vi "Quick Usb Write Setting.vi"(8 "error in (no error)":errorcluster, 9 "value":u16, 10 "address":u16, 11 "hDevice":u32) -> (0 "error out":errorcluster, 2 "function return":i32, 3 "hDevice out":u32)   [LabVIEW 2011, in "QuickUSB.lvlib"]
doc: "QUSBLIB QRETURN QuickUsbWriteSetting(\n QHANDLE hDevice,\n QWORD address, \n QWORD value\n);"
uses:
  QuickUSB.lvlib
  QuickUSB.dll
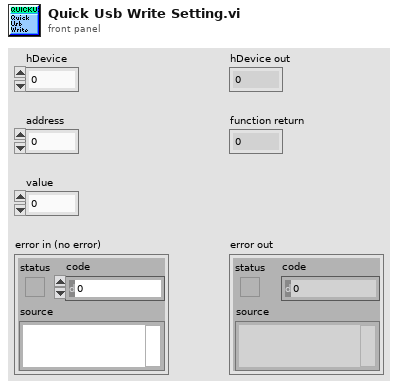
[diagram p1: front panel]
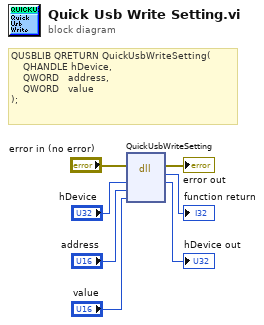
[diagram p0: block diagram]
diagram:
  # "QUSBLIB QRETURN QuickUsbWriteSetting(\n    QHANDLE hDevice,\n    QWORD   address, \n    QWORD   value\n);"
  n1 = dll-call lib="C:/QuickUSB/QuickUSB.*" fn="QuickUsbWriteSetting"(error in="error in (no error)", "hDevice"="hDevice", "address"="address", "value"="value") -> (error out=→"error out":errorcluster, →"function return":i32, "hDevice"=→"hDevice out":u32)  [unwired: 4 in, 1 out]
